vi "swap.vi"(8 "error in (no error)":errorcluster caption="错误输入（无错误）", 9 "j":u32, 10 "i":u32, 11 "MotorSystem 输入":refnum<class "MotorSystem.lvclass">) -> (0 "error out":errorcluster caption="错误输出", 3 "MotorSystem 输出":refnum<class "MotorSystem.lvclass">)   [LabVIEW 2016, in "MotionControl.lvlib" / "MotorSystem.lvclass"]
uses:
  <userlib>/MotionControl/MotorSystem/MotorSystem.lvclass
  <userlib>/MotionControl/MotorSystem/MotorSystem.lvclass/MotorSystem.ctl
  <userlib>/MotionControl/OneMotion/OneMotion.lvclass
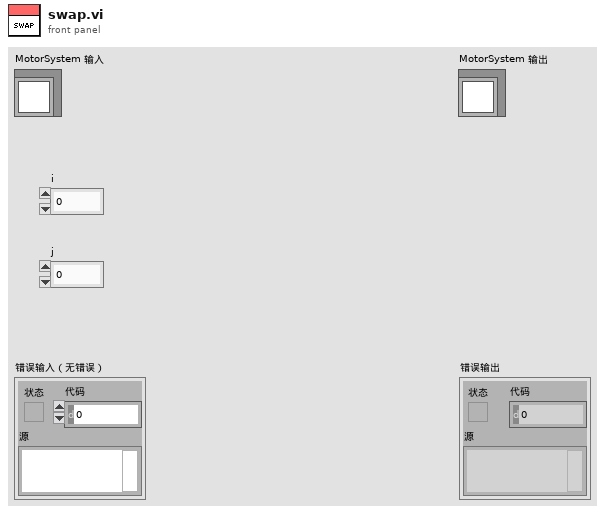
[diagram p1: front panel]
types:
  T1 = typedef "MotionControl.lvlib/MotorSystem.lvclass/MotionCluster.ctl" = cluster{"OneMotion.lvclass":refnum<class "OneMotion.lvclass">, "connected?":bool, "default enabled?":bool, "enabled?":bool}
  T2 = typedef "MotionControl.lvlib/StepMotor.lvclass/DEV_INFO.ctl" = cluster{"设备类型(0x01 = RS232CAN;0x02 = WIFI2RS232CAN;0x04 = USBCAN)":u32, "设备编号":u32, "系统为RS232CAN网关设备分配的COM口编号，这个成员变量只对\nRS232网关设备有用":u32, "RS232CAN网关设备与PC通讯的串口波特率，这个成员变量只对\nRS232网关设备有用":u32, "保存网关设备的名称":string}
  T3 = cluster{"complete dimension names":string[], "dimension names cluster ":cluster{"name 1":string, "name 2":string}}
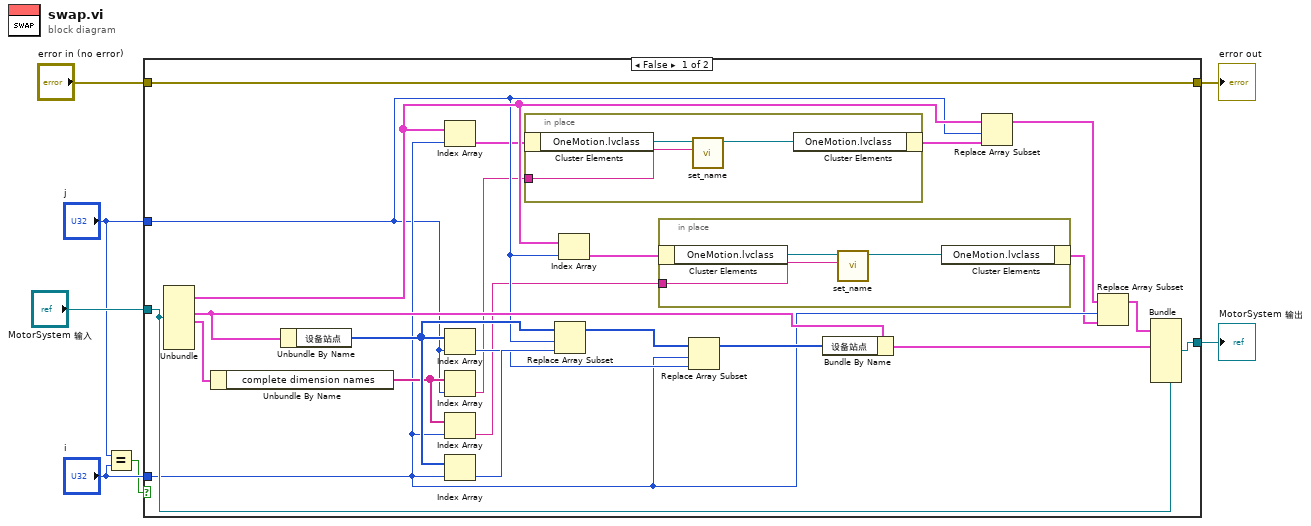
[diagram p0: block diagram]
diagram:
  n1 = Equal?(x="j", y="i") -> (x = y?=w1:bool)
  n2 = case shown="False" w1 {
    tunnel: [w30 w38] -> w7
    tunnel: [w18 w37] -> w5
    tunnel: "MotorSystem 输入" -> [w29 w37]
    tunnel: "error in (no error)" -> [w30 w38]
    tunnel: "i" -> [w15 _]
    tunnel: "j" -> [w14 _]
    frame False {
      n3 = Unbundle(w29) -> (w28:T1[], w21:cluster{"CAN 波特率":u32, "设备信息":T2, "设备站点":u32[]}, w17:T3)  [unwired: 5 out]
      n4 = Unbundle By Name(w17) -> ("complete dimension names"=w16:string[])
      n5 = Unbundle By Name(w21) -> ("设备站点"=w25:u32[])
      n6 = Index Array(array=w28, index=w15) -> (element=w13:T1)
      n7 = Index Array(array=w25, index=w14) -> (element=w22:u32)
      n8 = Index Array(array=w16, index=w14) -> (element=w11:string)
      n9 = Index Array(array=w16, index=w15) -> (element=w10:string)
      n10 = Index Array(array=w25, index=w15) -> (element=w23:u32)
      n11 = in-place {
        in-place-border: w11 -> [w34]
        n12 = in-place-cluster #1(w13) -> ("OneMotion.lvclass"=w36:refnum<class "OneMotion.lvclass">)
        n13 = call-dynamic "set_name.vi"("name"=w34, "OneMotion输入"=w36) -> ("OneMotion输出"=w35:refnum<class "OneMotion.lvclass">)  [unwired: 8 in, 1 out]
        n14 = in-place-cluster #1("OneMotion.lvclass"=w35) -> (w12:T1)
      }
      n15 = Replace Array Subset(array=w25, new element=w23, index=w14) -> (w24:u32[])
      n16 = Index Array(array=w28, index=w14) -> (element=w9:T1)
      n17 = in-place {
        in-place-border: w10 -> [w31]
        n18 = in-place-cluster #2(w9) -> ("OneMotion.lvclass"=w33:refnum<class "OneMotion.lvclass">)
        n19 = call-dynamic "set_name.vi"("name"=w31, "OneMotion输入"=w33) -> ("OneMotion输出"=w32:refnum<class "OneMotion.lvclass">)  [unwired: 8 in, 1 out]
        n20 = in-place-cluster #2("OneMotion.lvclass"=w32) -> (w8:T1)
      }
      n21 = Replace Array Subset(array=w24, new element=w22, index=w15) -> (w20:u32[])
      n22 = Bundle By Name(cluster=w21, "设备站点"=w20) -> (w19:cluster{"CAN 波特率":u32, "设备信息":T2, "设备站点":u32[]})
      n23 = Replace Array Subset(array=w28, new element=w12, index=w14) -> (w27:T1[])
      n24 = Replace Array Subset(array=w27, new element=w8, index=w15) -> (w26:T1[])
      n25 = Bundle(cluster=w29, w26, w19) -> (w18:refnum<class "MotorSystem.lvclass">)  [unwired: 6 in]
    }
    frame True {
    }
  }
  "error out" <- w7
  "MotorSystem 输出" <- w5
